vi "SRG_Query.vi"(0 "System no.":i32=1 min=1 max=4 step=1, 2 "Axes to query":string[](array[string]), 3 "Register no.":i32[](array[numeric]), 4 "Query all?":bool, 5 "error in":errorcluster) -> (14 "Register value":i32[](array[numeric]), 15 "Register value hex.":u32[](array[numeric]) format="%.0x", 19 "error out":errorcluster)   [LabVIEW 2020]
doc: "Returns register values for queried axes and register numbers. See motion processor or controller user manual for a description of bit-coded answer. If Query all? Is TRUE, Axes to query and Register no. are ignored and command is sent without any parameters to query all register numbers for all axes. \n\nC-843, C-843.PM: Register numbers are:\n- 1: Event status register\n- 2: Activity status register\n- 3: Signal status register\n\nC-866: Register numbers are:\n- 1: Event status register\n- 2: Activity status register\n- 3: Signal status register\n- 4: Signal sense\n\nC-413, C-867, C-877, C-884, C-885, C-891, E-135, E-712, E-754, E-861, E-871, E-873, E-874, Hydra, Pollux, Mercury, Mercury_GCS: Register number is:\n- 1: Status register"
uses:
  Global1.vi
panel:
  # "Returns register values for queried axes and register numbers."
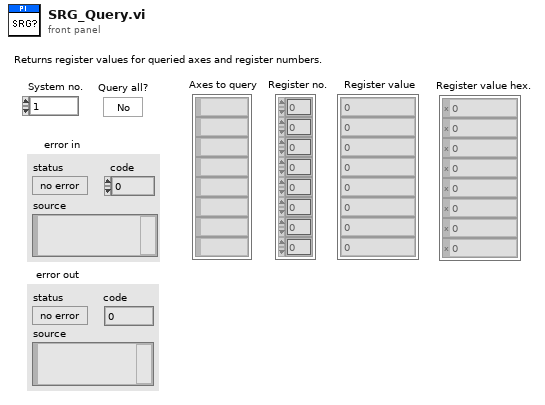
[diagram p1: front panel]
types:
  T1 = typedef "Syntax.ctl" = enum16{"GCS 1.0", "GCS 2.0", "GCS 3.0"}
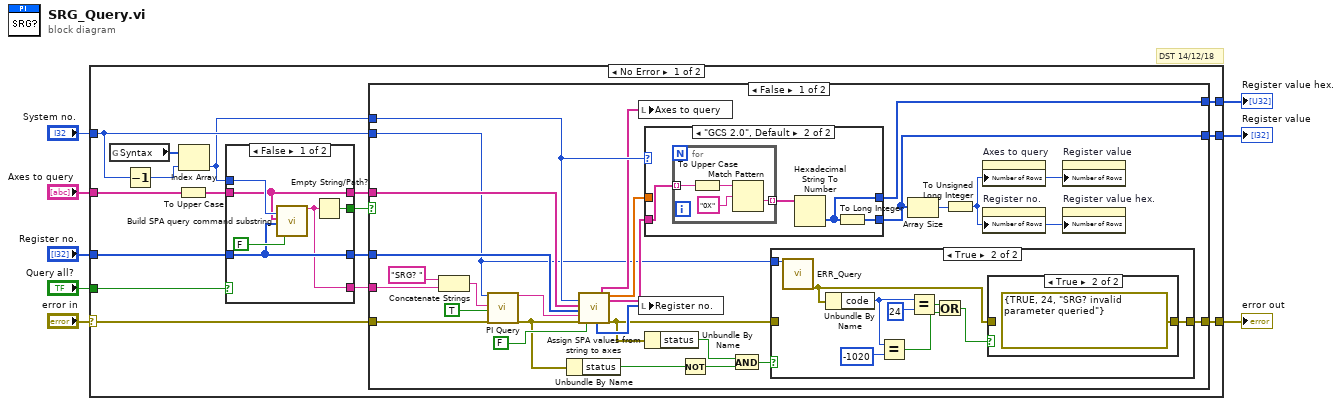
[diagram p0: block diagram]
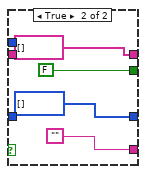
[diagram p2: hidden frame]
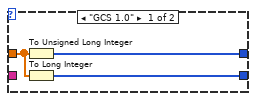
[diagram p3: hidden frame]
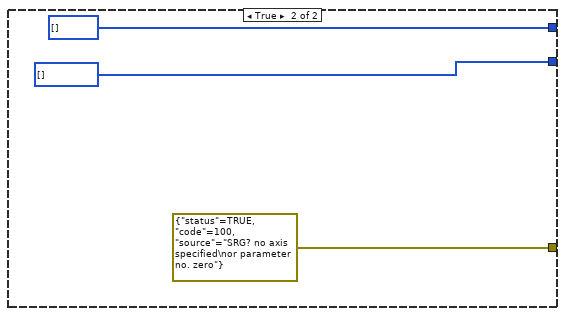
[diagram p6: hidden frame]
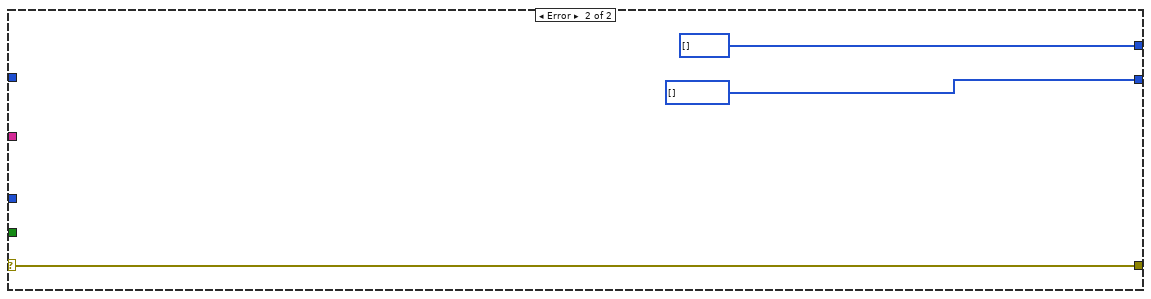
[diagram p7: hidden frame]
diagram:
  # "DST 14/12/18"
  n1 = case shown="No Error" "error in" {
    selector: "error in" -> [w9 w87]
    tunnel: "Axes to query" -> [w24 _]
    tunnel: "System no." -> [w16 _]
    tunnel: "Register no." -> [w21 _]
    tunnel: [w20 w87] -> w5
    tunnel: [w14 i32[] [] ("Parameter values")] -> w4
    tunnel: [w13 u32[] [] ("Parameter values")] -> w3
    tunnel: "Query all?" -> [w12 _]
    frame No Error {
      n2 = global read "Global1.vi" "Syntax"() -> (w17:T1[])
      n3 = Decrement(x=w16) -> (x-1=w18:i32)
      n4 = To Upper Case(1:w24) -> (0:w22:string[])
      n5 = Index Array(array=w17, index=w18) -> (element=w15:T1)
      n6 = case shown="False" w12 {
        tunnel: [w26 "" ("Command substring")] -> w23
        tunnel: w22 -> [w28 _]
        tunnel: w21 -> [w27 _]
        tunnel: [w25 FALSE] -> w19
        tunnel: w15 -> [w30 _]
        tunnel: [w28 string[] []] -> w11
        tunnel: [w27 i32[] [] ("Register no.")] -> w10
        frame False {
          n7 = call "Build SPA query command substring.vi"("Syntax"=w30, "Axes to query"=w28, "Parameter number"=w27, "Parameter no. format \n(Decimal: FALSE)"=FALSE ("Parameter no. format \n(Decimal: FALSE)")) -> ("Command substring"=w26:string)  [unwired: 3 in, 12 out]
          n8 = Empty String/Path?(string/path=w26) -> (empty?=w25:bool)
        }
        frame True {
        }
      }
      n9 = case shown="False" w19 {
        tunnel: w9 -> [w46 _]
        tunnel: w23 -> [w57 _]
        tunnel: w11 -> [w56 _]
        tunnel: w16 -> [w40 _]
        tunnel: w10 -> [w55 _]
        tunnel: [w52 errorcluster {"status"=TRUE, "code"=100, "source"="SRG? no axis specified\nor parameter no. zero"} ("error out")] -> w20
        tunnel: [w45 i32[] [] ("Parameter values")] -> w14
        tunnel: w15 -> [w50 _]
        tunnel: [w47 u32[] []] -> w13
        frame False {
          n10 = Concatenate Strings("SRG? ", w57) -> (w58:string)
          n11 = call "PI Query.vi"("System no."=w40, "String to send"=w58, "Attach termination char.?"=TRUE ("Attach Linefeed?"), "error in"=w46) -> ("String read"=w41:string, "error out"=w38:errorcluster)  [unwired: 3 in, 11 out]
          n12 = Unbundle By Name(w38) -> ("status"=w36:bool)
          n13 = call "Assign SPA values from string to axes.vi"("Syntax"=w50, "Queried axes"=w56, "Parameter no."=w55, "Input string"=w41, "error in"=w38, "Parameter no. format \n(Decimal: FALSE)"=FALSE ("Parameter no. format \n(Decimal: FALSE)")) -> ("Parameter no. out"=w42:i32[], "Queried axes out"=w43:string[], "Parameter values"=w49:dbl[], "Parameter strings"=w48:string[], "error out"=w39:errorcluster)  [unwired: 2 in, 7 out]
          n14 = local write "Axes to query"(w43) -> ()
          n15 = local write "Register no."(w42) -> ()
          n16 = case shown="\"GCS 2.0\", Default" w50 {
            tunnel: w49 -> [w62 _]
            tunnel: [w63 w64] -> w45
            tunnel: w48 -> [_ w67]
            tunnel: [w61 w65] -> w47
            frame "GCS 1.0" {
              n17 = To Unsigned Long Integer(number=w62) -> (unsigned 32bit integer=w61:u32[])
              n18 = To Long Integer(number=w62) -> (32bit integer=w63:i32[])
            }
            frame "GCS 2.0", Default {
              n19 = for {
                tunnel: w67 -> [w69] mode=indexing
                tunnel: [w68] -> w66 mode=indexing
                n20 = To Upper Case(1:w69) -> (0:w70:string)
                n21 = Match Pattern(string=w70, regular expression="0X") -> (after substring=w68:string)  [unwired: 4 out]
              }
              n22 = Hexadecimal String To Number(string=w66) -> (number=w65:u32[])  [unwired: 3 out]
              n23 = To Long Integer(number=w65) -> (32bit integer=w64:i32[])
            }
          }
          n24 = Unbundle By Name(w39) -> ("status"=w54:bool)
          n25 = Not(x=w36) -> (.not. x?=w37:bool)
          n26 = And(x=w54, y=w37) -> (x .and. y?=w53:bool)
          n27 = case shown="True" w53 {
            tunnel: w39 -> [w72 _]
            tunnel: [w72 w74] -> w52
            tunnel: w40 -> [_ w81]
            frame False {
            }
            frame True {
              n28 = call "ERR_Query.vi"("System no."=w81) -> ("error out"=w73:errorcluster)  [unwired: 1 in, 17 out]
              n29 = Unbundle By Name(w73) -> ("code"=w78:i32)
              n30 = Equal?(x=w78, y=-1020) -> (x = y?=w76:bool)
              n31 = Equal?(x=w78, y=24) -> (x = y?=w77:bool)
              n32 = Or(x=w77, y=w76) -> (x .or. y?=w75:bool)
              n33 = case shown="True" w75 {
                tunnel: [w82 errorcluster {TRUE, 24, "SRG? invalid parameter queried"} ("output cluster")] -> w74
                tunnel: w73 -> [w82 _]
                frame False {
                }
                frame True {
                }
              }
            }
          }
          n34 = Array Size(array=w45) -> (size(s)=w44:i32)
          n35 = To Unsigned Long Integer(number=w44) -> (unsigned 32bit integer=w35:u32)
          n36 = property on="Axes to query" class="Arr (strict)"("Number of Rows"=w35) -> ()  [unwired: 2 in, 2 out]
          n37 = property on="Register no." class="Arr (strict)"("Number of Rows"=w35) -> ()  [unwired: 2 in, 2 out]
          n38 = property on="Register value" class="Arr (strict)"("Number of Rows"=w35) -> ()  [unwired: 2 in, 2 out]
          n39 = property on="Register value hex." class="Arr (strict)"("Number of Rows"=w35) -> ()  [unwired: 2 in, 2 out]
        }
        frame True {
        }
      }
    }
    frame Error {
    }
  }
  "error out" <- w5
  "Register value" <- w4
  "Register value hex." <- w3
